vi "Untitled1.vi"() -> ()   [LabVIEW 2024]
uses:
  <vilib>/Platform/TimedLoop/XDataNode/timing_clust.ctl
  <vilib>/Platform/TimedLoop/XDataNode/nitl_modes.ctl
  <vilib>/Platform/TimedLoop/XDataNode/wakeup.ctl
  <vilib>/DAQmx/read.llb/DAQmx Read (Analog 1D Wfm NChan 1Samp).vi
  <vilib>/DAQmx/read.llb/DAQmx Read (Analog 1D DBL NChan 1Samp).vi
  <vilib>/DAQmx/create/channels.llb/DAQmx Create Channel (AI-Voltage-Basic).vi
  <vilib>/DAQmx/miscellaneous.llb/DAQmx Fill In Error Info.vi
  <vilib>/platform/TimedLoop/XDataNode/XDataNode.xnode
  <vilib>/Platform/TimedLoop/XDataNode/XDNodeRunTimeDep.lvlib
panel:
  in  "HWSerialNum":i32
  in  "MG17Motor":refnum<k7>(container)
  out "Waveform Chart":sgl(graph)
  out "pfPosition":sgl
  out "data":waveform(dbl)[](array[waveform])
  out "output cluster":cluster{"Waveform":dbl}
  out "error out":errorcluster
  out "Waveform Chart 2":dynamicdata(graph)
  in  "DAQmx Physical Channel":tag
  in  "stop":bool
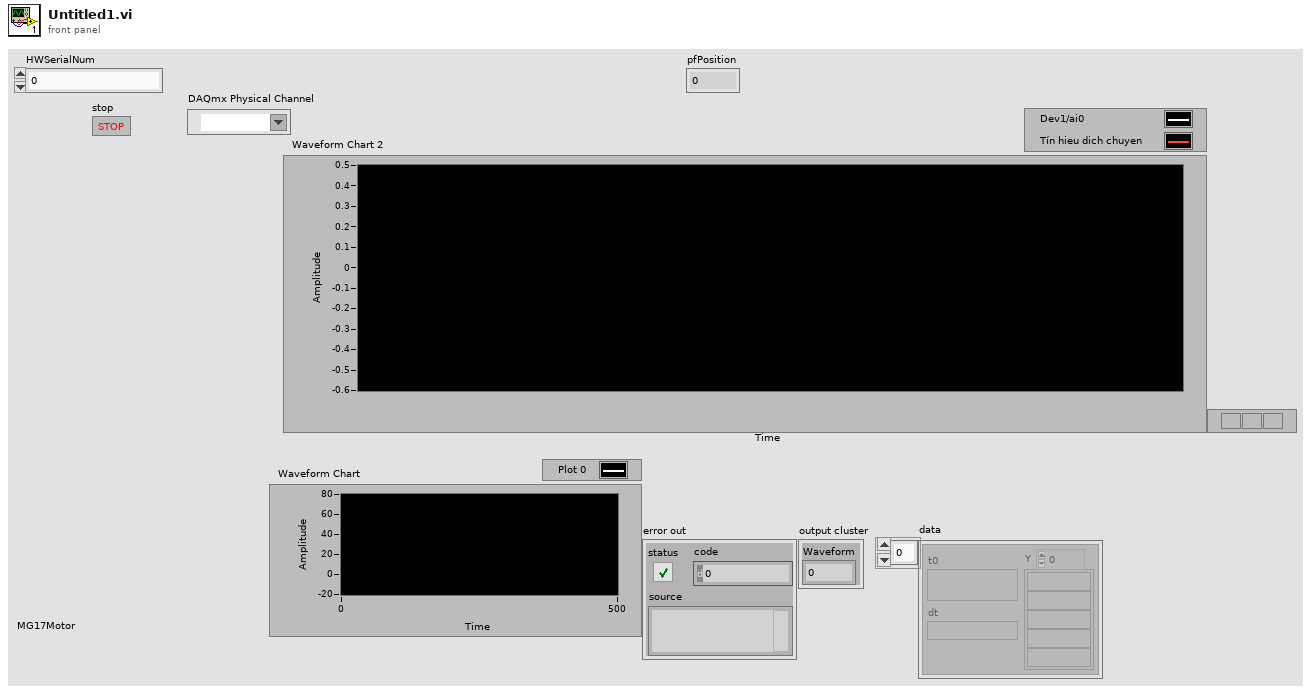
[diagram p1: front panel]
types:
  T1 = typedef "XDNodeRunTimeDep.lvlib/timing_clust.ctl" = cluster{"Expected End [f-1]":u64, "Actual End [f-1]":u64, "Finished Late? [f-1]":bool, "Expected End [i-1]":u64, "Actual End [i-1]":u64, "Finished Late? [i-1]":bool, "Expected Start [i]":u64, "Actual Start [i]":u64, "Expected Start [f]":u64, "Actual Start [f]":u64, "Source Name":string, "Structure Name":string, "Period":i64, "Deadline":i64, "Offset":i64, "Start":i64, "Priority":i32, "Timeout":i32, "Mode":T2, "Wakeup Reason":T3, "Error":errorcluster, "Source Type":string, "Secondary Source Type":string, "Global End Time":u64, "Global Start Time":u64, "Frame Duration":u64, "Iteration Duration":u64, "Assigned CPU":i32, "I/O Scan Engine Mode":u32}
  T2 = typedef "XDNodeRunTimeDep.lvlib/nitl_modes.ctl" = enum32{"No Change", "Process missed periods, maintain original phase", "Discard missed periods, maintain original phase", "Process missed periods, ignore original phase", "Discard missed periods, ignore original phase"}
  T3 = typedef "XDNodeRunTimeDep.lvlib/wakeup.ctl" = enum32{"Normal", "Aborted", "Asynchronous wakeup", "Timing source error", "Timed loop error", "Timeout"}
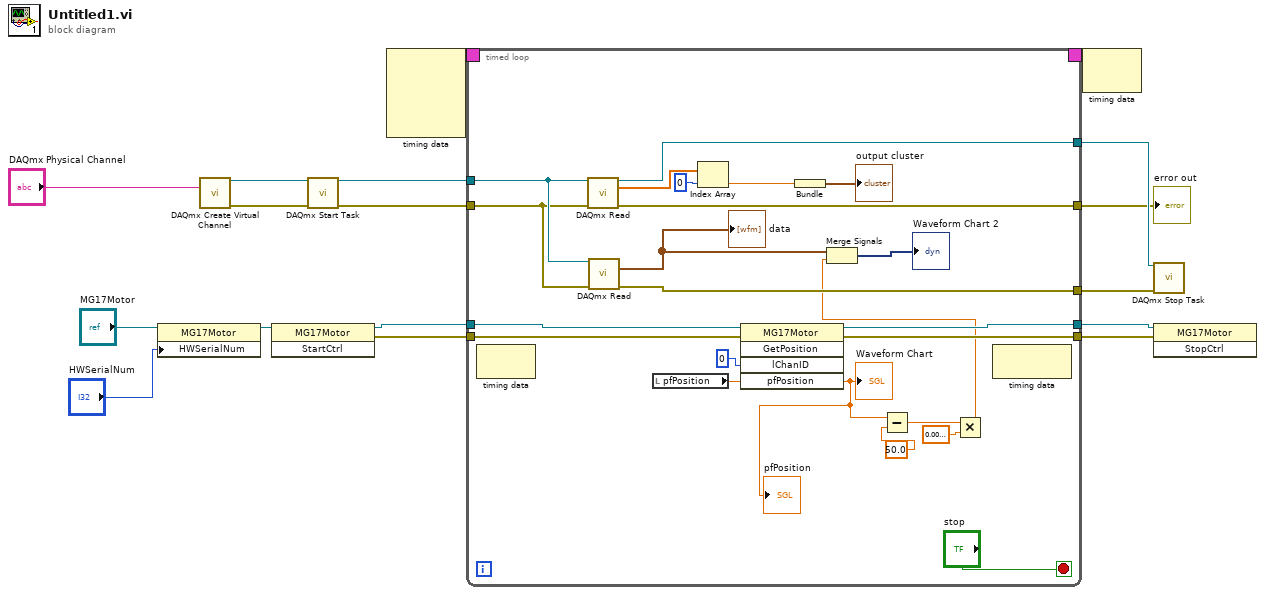
[diagram p0: block diagram]
diagram:
  n1 = property class="MG17Motor"(reference="MG17Motor", "HWSerialNum"="HWSerialNum") -> (reference out=w5:refnum<k7>)  [unwired: 1 in, 1 out]
  n2 = call-poly <vilib>:"DAQmx Create Virtual Channel.vi"("physical channels"="DAQmx Physical Channel") -> ("task out"=w15:refnum<k21>, "error out"=w12:errorcluster)  [unwired: 13 in]
  n3 = invoke class="MG17Motor" method="StartCtrl"(reference=w5) -> (reference out=w4:refnum<k7>, error out=w3:errorcluster)  [unwired: 2 in, 1 out]
  n4 = call <vilib>:"DAQmx Start Task.vi"("task/channels in"=w15, "error in"=w12) -> ("task out"=w14:refnum<k21>, "error out"=w11:errorcluster)  [unwired: 12 in]
  n5 = node-c288() -> (w17:T1)  [unwired: 4 in]
  n6 = timed-loop {
    timing: w17 -> [_]
    timing-out: [_] -> w16
    tunnel: w14 -> [w35]
    tunnel: [w39] -> w13
    tunnel: w11 -> [w34]
    tunnel: [w33] -> w10
    tunnel: [w32] -> w8
    tunnel: w4 -> [w23]
    tunnel: w3 -> [w22]
    tunnel: [w21] -> w2
    tunnel: [w20] -> w1
    stop <- "stop" stop-if-true
    n7 = node-c288() -> ()  [unwired: 1 in, 1 out]
    n8 = call-poly <vilib>:"DAQmx Read.vi"("task/channels in"=w35, "error in"=w34) -> ("task out"=w39:refnum<k21>, "data"=w38:dbl[], "error out"=w32:errorcluster)  [unwired: 11 in]
    n9 = call-poly <vilib>:"DAQmx Read.vi"("task/channels in"=w35, "error in"=w34) -> ("data"=w29:waveform(dbl)[], "error out"=w33:errorcluster)  [unwired: 11 in, 1 out]
    "data" <- w29
    n10 = local read "pfPosition"() -> (w25:sgl)
    n11 = Index Array(array=w38, index=0) -> (element=w36:dbl)
    n12 = invoke class="MG17Motor" method="GetPosition"(reference=w23, error in=w22, "lChanID"=0, "pfPosition"=w25) -> (reference out=w21:refnum<k7>, error out=w20:errorcluster, "pfPosition"=w19:sgl)  [unwired: 1 in, 2 out]
    "pfPosition" <- w19
    "Waveform Chart" <- w19
    n13 = Bundle("Waveform"=w36) -> (→"output cluster":cluster{"Waveform":dbl})  [unwired: 1 in]
    n14 = Subtract(x=w19, y=sgl 50.0) -> (x-y=w24:sgl)
    n15 = Multiply(x=w24, y=sgl 0.01 ("x")) -> (x*y=w18:sgl)
    n16 = Merge Signals(w29, w18) -> (→"Waveform Chart 2":dynamicdata)
    n17 = node-c288() -> ()  [unwired: 1 in, 1 out]
  }
  "error out" <- w8
  n18 = node-c288(w16) -> ()  [unwired: 1 out]
  n19 = call <vilib>:"DAQmx Stop Task.vi"("task/channels in"=w13, "error in"=w10) -> ()  [unwired: 12 in, 2 out]
  n20 = invoke class="MG17Motor" method="StopCtrl"(reference=w2, error in=w1) -> ()  [unwired: 1 in, 3 out]
